vi "Stop Application.vi"(8 "error in (no error)":errorcluster, 11 "Channel Manager in":refnum<class "Channel Manager.lvclass">) -> (0 "error out":errorcluster, 2 "Stop Application":bool, 3 "Channel Manager out":refnum<class "Channel Manager.lvclass">)   [LabVIEW 2018, in "Channel Manager.lvclass"]
uses:
  Channel Manager.lvclass
  Channel Manager.lvclass/Channel Manager.ctl
  Channel/Channel.lvclass
  RxTx/RxTx.lvclass
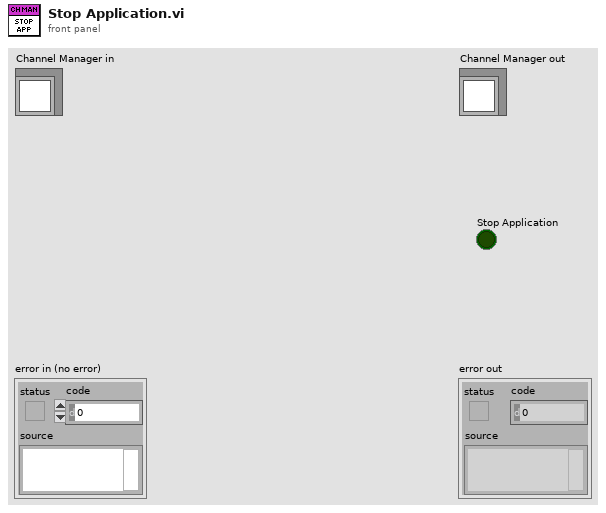
[diagram p1: front panel]
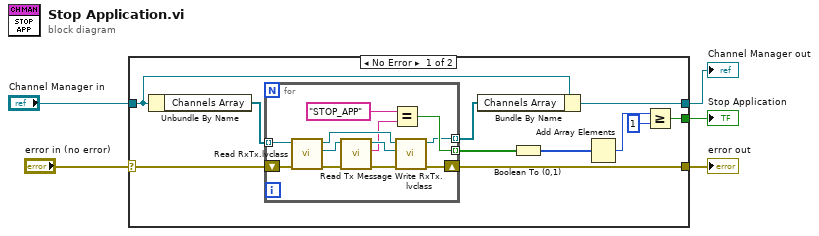
[diagram p0: block diagram]
diagram:
  n1 = case shown="No Error" "error in (no error)" {
    selector: "error in (no error)" -> [w15 w30]
    tunnel: [w9 w30] -> w4
    tunnel: [w7 w29] -> w2
    tunnel: "Channel Manager in" -> [w8 w29]
    tunnel: [w10 _] -> w1
    frame No Error {
      n2 = Unbundle By Name(w8) -> ("Channels Array"=w16:refnum<class "Channel.lvclass">[])
      n3 = for {
        tunnel: w16 -> [w17] mode=indexing
        tunnel: [w27] -> w14 mode=indexing
        shift-right: [w19] -> w9
        shift-left: w15 -> [w18]
        tunnel: [w20] -> w6 mode=indexing
        n4 = call "Read RxTx.lvclass.vi"("error in (no error)"=w18, "Channel in"=w17) -> ("error out"=w23:errorcluster, "RxTx.lvclass"=w26:refnum<class "RxTx.lvclass">, "Channel out"=w24:refnum<class "Channel.lvclass">)  [unwired: 7 in]
        n5 = call "Read Tx Message.vi"("error in (no error)"=w23, "RxTx in"=w26) -> ("error out"=w22:errorcluster, "Tx Message"=w21:string, "RxTx out"=w25:refnum<class "RxTx.lvclass">)  [unwired: 7 in]
        n6 = Equal?(x="STOP_APP", y=w21) -> (x = y?=w27:bool)
        n7 = call "Write RxTx.lvclass.vi"("error in (no error)"=w22, "RxTx.lvclass"=w25, "Channel in"=w24) -> ("error out"=w19:errorcluster, "Channel out"=w20:refnum<class "Channel.lvclass">)  [unwired: 7 in]
      }
      n8 = Bundle By Name(cluster=w8, "Channels Array"=w6) -> (w7:refnum<class "Channel Manager.lvclass">)
      n9 = Boolean To (0,1)(Boolean=w14) -> (0, 1=w13:i16[])
      n10 = Add Array Elements(numeric array=w13) -> (sum=w12:i16)
      n11 = Greater Or Equal?(x=w12, y=i16 1) -> (x >= y?=w10:bool)
    }
    frame Error {
    }
  }
  "error out" <- w4
  "Channel Manager out" <- w2
  "Stop Application" <- w1
